vi "Plot 3D Polynomial Fit.vi"(6 "Coefficients":dbl[](array[numeric]) format="%.3e", 7 "Highest order":i32=1, 8 "error in":errorcluster, 9 "Z":dbl[](array[numeric]), 10 "Y":dbl[](array[numeric]), 11 "X":dbl[](array[numeric])) -> (0 "error out":errorcluster, 3 "3D Graph":refnum<class "Base Datatype.lvclass">[](array[class]))   [LabVIEW 2013]
doc: "This .vi plots the data and fit on the same 3D Plot. Copy the 3D Plot control from \"3D Polynomial Fit.vi\" to start with a nice looking graph."
uses:
  <vilib>/Native 3D Graph/classes/Base Datatype.lvclass
  <vilib>/Analysis/1siggen.llb/Ramp Pattern by Samples.vi
  <vilib>/Native 3D Graph/xcontrol/3DPC_SurfacePlot.xctl
  <vilib>/Analysis/NI_AALBase.lvlib
panel:
  # "Copy the 3D Plot control from \"3D Polynomial Fit.vi\" to start with a nice looking graph."
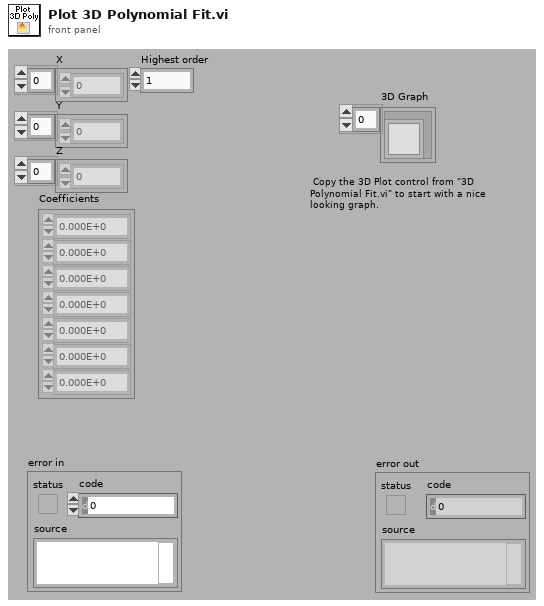
[diagram p1: front panel]
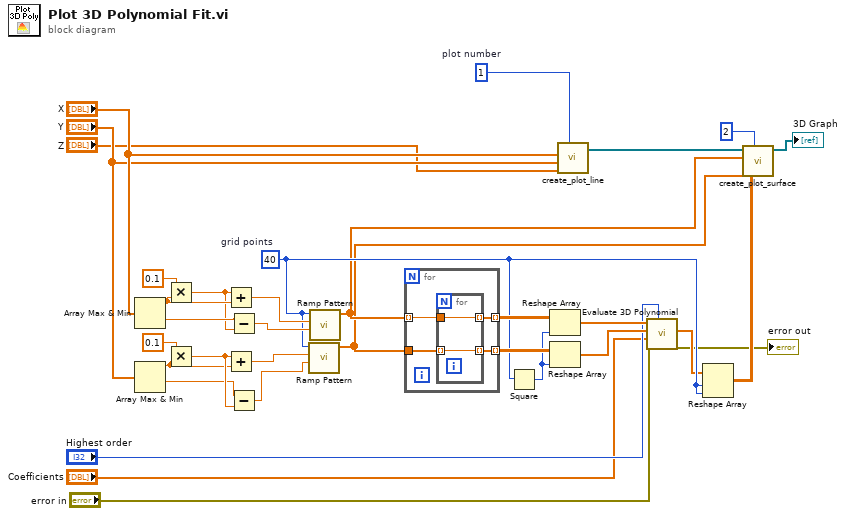
[diagram p0: block diagram]
diagram:
  w3 = 1  # plot number
  w19 = 40  # grid points
  n1 = Array Max & Min(array="X") -> (max value=w30:dbl, min value=w29:dbl)  [unwired: 2 out]
  n2 = Array Max & Min(array="Y") -> (max value=w23:dbl, min value=w24:dbl)  [unwired: 2 out]
  n3 = Multiply(x=0.1, y=w30) -> (x*y=w28:dbl)
  n4 = Multiply(x=0.1, y=w23) -> (x*y=w25:dbl)
  n5 = Add(x=w28, y=w30) -> (x+y=w26:dbl)
  n6 = Add(x=w25, y=w23) -> (x+y=w21:dbl)
  n7 = Subtract(x=w29, y=w28) -> (x-y=w27:dbl)
  n8 = Subtract(x=w24, y=w25) -> (x-y=w20:dbl)
  n9 = call-poly <vilib>:"Ramp Pattern.vi"("start"=w20, "end"=w21, "samples"=w19) -> ("Ramp Pattern"=w9:dbl[])  [unwired: 7 in, 1 out]
  n10 = call-poly <vilib>:"Ramp Pattern.vi"("start"=w27, "end"=w26, "samples"=w19) -> ("Ramp Pattern"=w10:dbl[])  [unwired: 7 in, 1 out]
  n11 = for {
    tunnel: w10 -> [w37] mode=indexing
    tunnel: w9 -> [w36]
    tunnel: [w35] -> w32 mode=indexing
    tunnel: [w34] -> w33 mode=indexing
    n12 = for {
      tunnel: w37 -> [w39]
      tunnel: w36 -> [w38] mode=indexing
      tunnel: [w39] -> w35 mode=indexing
      tunnel: [w38] -> w34 mode=indexing
    }
  }
  n13 = Square(x=w19) -> (x^2=w18:i32)
  n14 = Reshape Array(w32, w18) -> (w16:dbl[])
  n15 = Reshape Array(w33, w18) -> (w17:dbl[])
  n16 = call <vilib>:"create_plot_line.vi"("plot ID"=w3, "z vector"="Z", "y vector"="Y", "x vector"="X") -> ("plots out"=w7:refnum<class "Base Datatype.lvclass">[])  [unwired: 1 in, 6 out]
  n17 = call "Evaluate 3D Polynomial.vi"("Highest order"="Highest order", "error in"="error in", "Coefficients"="Coefficients", "Y"=w17, "X"=w16) -> ("error out"=→"error out":errorcluster, "Z"=w15:dbl[])  [unwired: 5 out]
  n18 = Reshape Array(w15, w19, w19) -> (w12:dbl[][])
  n19 = call <vilib>:"create_plot_surface.vi"("plot ID"=2 ("Plot ID"), "z matrix"=w12, "y vector"=w9, "x vector"=w10, "plots in"=w7) -> ("plots out"=→"3D Graph":refnum<class "Base Datatype.lvclass">[])  [unwired: 1 in, 5 out]
